vi "PantherLAB_Log - Rename DQMH Module.vi"(9 "New Module Library":path, 10 "Module Info (old)":T1, 11 "Project":refnum<vi>) -> (0 "error out":errorcluster)   [LabVIEW 2016]
doc: "_____\nCreated using DQMH Framework: Event Scripter 7.1.0.1450."
uses:
  <vilib>/Delacor/Delacor QMH/Libraries/_Scripting Support/Module Info--cluster.ctl
  <vilib>/Delacor/Delacor QMH/Libraries/_Scripting Support/Module Type--enum.ctl
  PantherLAB Scripting Hooks/PantherLAB_Scripting.lvlib
  <vilib>/Delacor/Delacor QMH/Libraries/_Scripting Support/dqmh_lib_DQMH Scripting Support.lvlib
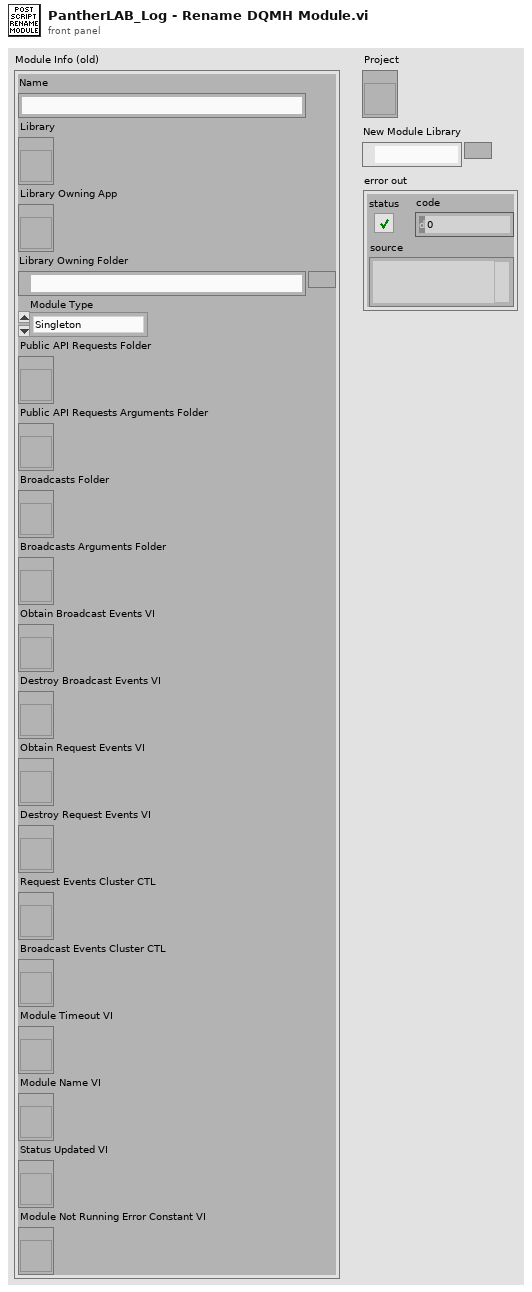
[diagram p1: front panel]
types:
  T1 = typedef "dqmh_lib_DQMH Scripting Support.lvlib/Module Info--cluster.ctl" = cluster{"Name":string, "Library":refnum<vi>, "Library Owning App":refnum<vi>, "Library Owning Folder":path, "Module Type":T2, "Public API Requests Folder":refnum<vi>, "Public API Requests Arguments Folder":refnum<vi>, "Broadcasts Folder":refnum<vi>, "Broadcasts Arguments Folder":refnum<vi>, "Obtain Broadcast Events VI":refnum<vi>, "Destroy Broadcast Events VI":refnum<vi>, "Obtain Request Events VI":refnum<vi>, "Destroy Request Events VI":refnum<vi>, "Request Events Cluster CTL":refnum<vi>, "Broadcast Events Cluster CTL":refnum<vi>, "Module Timeout VI":refnum<vi>, "Module Name VI":refnum<vi>, "Status Updated VI":refnum<vi>, "Module Not Running Error Constant VI":refnum<vi>}
  T2 = typedef "dqmh_lib_DQMH Scripting Support.lvlib/Module Type--enum.ctl" = enum16{"Singleton", "Cloneable"}
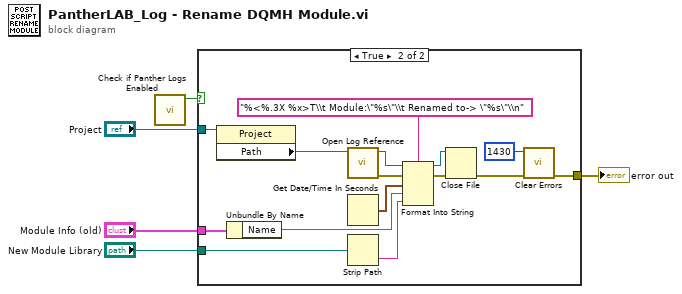
[diagram p0: block diagram]
diagram:
  n1 = call "Check if Panther Logs Enabled.vi"() -> ("PantherLogs Enabled?"=w4:bool)  [unwired: 11 in]
  n2 = case shown="True" w4 {
    tunnel: [_ w17] -> w5
    tunnel: "Project" -> [_ w13]
    tunnel: "Module Info (old)" -> [_ w11]
    tunnel: "New Module Library" -> [_ w10]
    frame False {
    }
    frame True {
      n3 = property class="Project"(reference=w13) -> ("Path"=w12:path)  [unwired: 1 in, 2 out]
      n4 = Unbundle By Name(w11) -> ("Name"=w9:string)
      n5 = call "Open Log Reference.vi"("Project Path"=w12) -> ("error out"=w20:errorcluster, "File Reference"=w16:refnum<file>)  [unwired: 9 in]
      n6 = Get Date/Time In Seconds() -> (seconds since 1Jan1904=w14:timestamp)
      n7 = Strip Path(path=w10) -> (name=w8:string)  [unwired: 1 out]
      n8 = Format Into String(format string="%<%.3X %x>T\\t Module:\"%s\"\\t Renamed to-> \"%s\"\\n", initial string=w16, error in=w20, w14, w9, w8) -> (resulting string=w15:refnum<file>, error out=w19:errorcluster)
      n9 = Close File(refnum=w15, error in=w19) -> (error out=w18:errorcluster)  [unwired: 1 out]
      n10 = call <vilib>:"Clear Errors.vi"("error in (no error)"=w18, "specific error code to clear (0: all)"=1430) -> ("error out"=w17:errorcluster)  [unwired: 4 in, 1 out]
    }
  }
  "error out" <- w5
